vi "Define_dR_Area_for_11_Displ-1.vi"(4 "[IN] Areas particles\nPrimary Detected":dbl[][](array[numeric]), 6 "[IN] Primary \n(X,Y) Detected":dbl[][](array[numeric]), 8 "error IN":errorcluster, 9 "[IN] Subtrack":T1, 11 "[IN] Still connect\ned tracks in group":T2) -> (0 "error OUT":errorcluster, 2 "[OUT] Area of  \"11\" \ndestination point":dbl, 3 "[OUT] dR for 11 \ndisplacement":dbl)   [LabVIEW 2013]
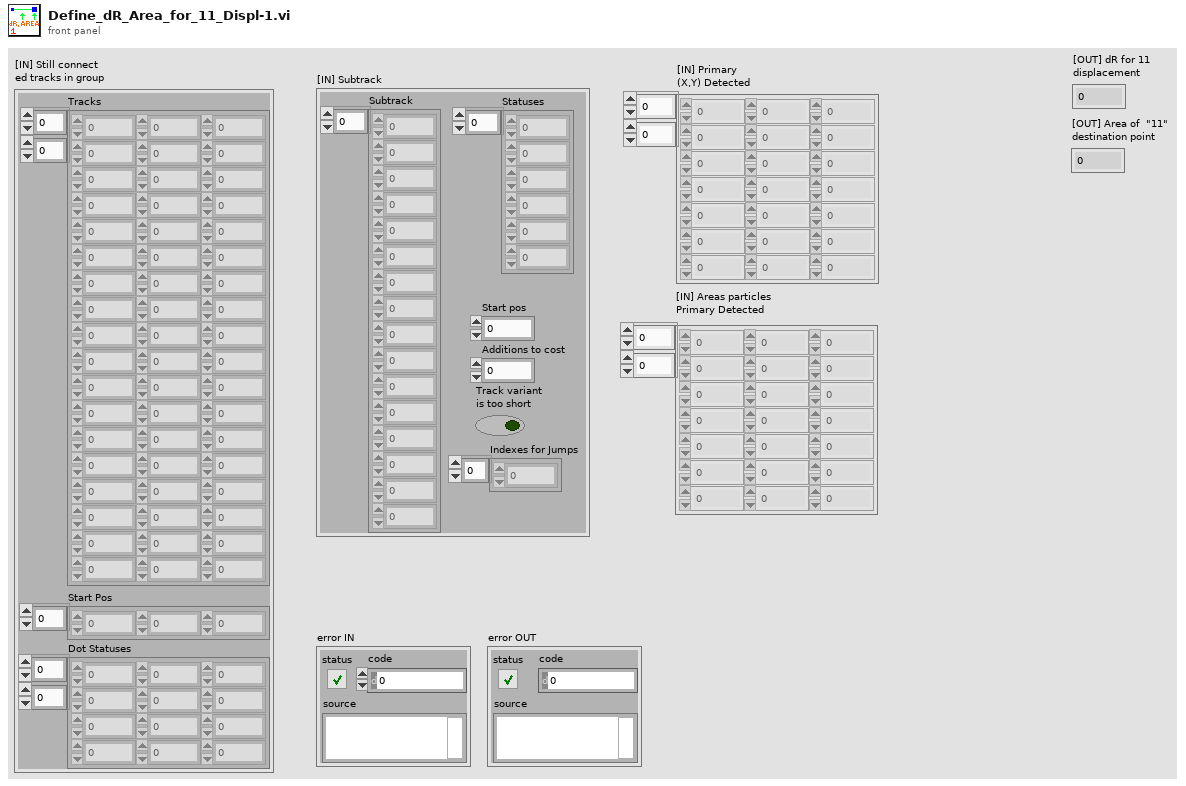
[diagram p1: front panel]
types:
  T1 = cluster{"Subtrack":dbl[], "Statuses":i16[], "Start pos":i32, "Additions to cost":i32, "Track variant \nis too short":bool, "Indexes for Jumps":i32[]}
  T2 = cluster{"Tracks":dbl[][], "Start Pos":i32[], "Dot Statuses":i16[][]}
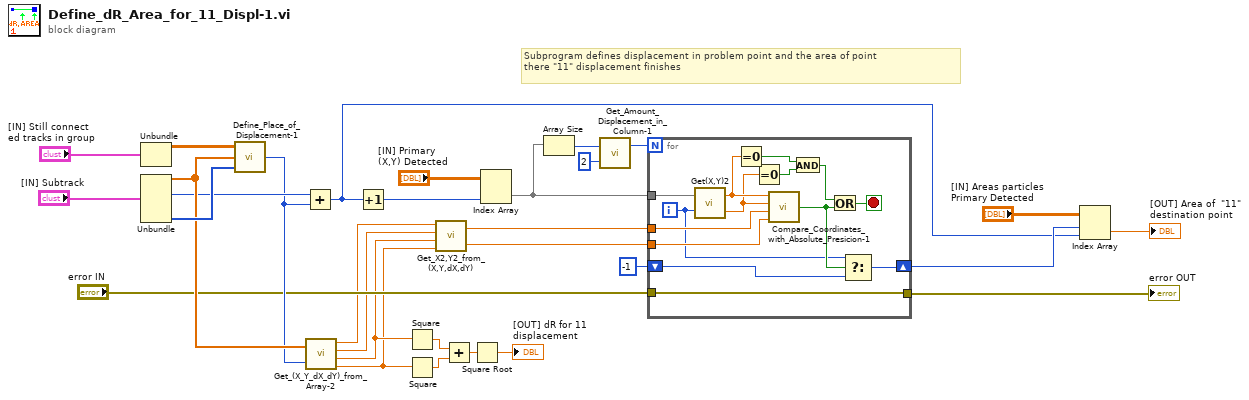
[diagram p0: block diagram]
diagram:
  # "Subprogram defines displacement in problem point and the area of point \nthere \"11\" displacement finishes"
  n1 = Unbundle("[IN] Still connect\ned tracks in group") -> ("Tracks"=w29:dbl[][])  [unwired: 2 out]
  n2 = Unbundle("[IN] Subtrack") -> ("Subtrack"=w23:dbl[], "Start pos"=w16:i32, "Indexes for Jumps"=w27:i32[])  [unwired: 3 out]
  n3 = call "Define_Place_of_Displacement-1.vi"("[IN] Indexes for Jumps"=w27, "[IN] Subtrack"=w23, "[IN] Tracks"=w29) -> ("[OUT] Index of \"11\" Dis\nplacement in Subtrack"=w15:i32)  [unwired: 2 in]
  n4 = Add(x=w16, y=w15) -> (x+y=w8:i32)
  n5 = call "Get_(X_Y_dX_dY)_from_Array-2.vi"("(X,Y,dX,dY)"=w23, "Index of Displacement"=w15) -> ("X"=w6:dbl, "Y"=w5:dbl, "dX"=w4:dbl, "dY"=w3:dbl)
  n6 = Increment(x=w8) -> (x+1=w7:i32)
  n7 = Square(x=w4) -> (x^2=w26:dbl)
  n8 = Square(x=w3) -> (x^2=w25:dbl)
  n9 = call "Get_X2,Y2_from_(X,Y,dX,dY).vi"("dY"=w3, "dX"=w4, "Y1"=w5, "X1"=w6) -> ("Y2 = (Y1+dY)"=w1:dbl, "X2 = (X1+dX)"=w2:dbl)
  n10 = Add(x=w26, y=w25) -> (x+y=w24:dbl)
  n11 = Square Root(x=w24) -> (sqrt(x)=→"[OUT] dR for 11 \ndisplacement":dbl)
  n12 = Index Array(array="[IN] Primary \n(X,Y) Detected", index (col)=w7) -> (element=w17:dbl[])  [unwired: 1 in]
  n13 = Array Size(array=w17) -> (size(s)=w21:i32)
  n14 = call "Get_Amount_Displacement_in_Column-1.vi"("multiplier"=2, "# Rows"=w21) -> ("Displ amount"=w19:i32)  [unwired: 1 out]
  n15 = for {
    N: w19 -> [_]
    tunnel: w17 -> [w43]
    tunnel: w2 -> [w42]
    tunnel: w1 -> [w41]
    shift-right: [w32] -> w10
    shift-left: -1 -> [w33]
    tunnel: "error IN" -> [w31]
    tunnel: [w31] -> w12
    i -> [w34]
    stop <- w44 stop-if-true
    n16 = call "Get(X,Y)2.vi"("[IN] index of (X,Y)"=w34, "[IN] Array coordi\nnates (X,Y) in Frame"=w43) -> ("[OUT] Y"=w37:dbl, "[OUT] X"=w38:dbl)
    n17 = Equal To 0?(x=w38) -> (x = 0?=w40:bool)
    n18 = Equal To 0?(x=w37) -> (x = 0?=w39:bool)
    n19 = call "Compare_Coordinates_with_Absolute_Presicion-1.vi"("X 1"=w38, "Y 1"=w37, "X 2"=w42, "Y 2"=w41) -> ("[OUT] Same coordinates?"=w35:bool)  [unwired: 1 in]
    n20 = And(x=w40, y=w39) -> (x .and. y?=w36:bool)
    n21 = Or(x=w36, y=w35) -> (x .or. y?=w44:bool)
    n22 = Select(t=w34, s=w35, f=w33) -> (s? t:f=w32:i32)
  }
  "error OUT" <- w12
  n23 = Index Array(array="[IN] Areas particles\nPrimary Detected", index (row)=w10, index (col)=w8) -> (element=→"[OUT] Area of  \"11\" \ndestination point":dbl)
